vi "Write_setup_to_BSA_F60.vi"(2 "No Of Samples":i32, 3 "Time (s)":sgl, 4 "BSA Setup In":T1={"Wavelength (nm)"=514.5, "Vel Comp"="W", "Max Velocity"=0.0, "Min Velocity"=0.0, "Max Record length"=2, "Signal gain (dB)"=30, "High voltage"=2000, "Optics Conversion Factor"=0.0, "Min Record length"=2, "Multiply Velocity by -1"=FALSE, "Signal to Noise Ratio"="0", "Validation Ratio"="4", "Probe"="", "Laser"="", "BSA"="", "Lense"="", "Beam Separation (mm)"=514.5, "Focal Length (mm)"=514.5, "COLOUR"=52224, "BSA IP"="", "Velocity Range (m/s)"=0.0, "Centre Velocity (m/s)"=0.0, "Unshifted mW"=0.0, "Shifted mW"=0.0, "Bandwidth Hz"=0.0, "Req Sampling Rate Hz"=100.0, "Ch"=0, "CenterFreq Hz"=0.0, "Laser IP"=""} {"Req Sampling Rate Hz" min=1.0; "Shifted mW" format="%.1g"; "Unshifted mW" format="%.1g"; "Centre Velocity (m/s)" format="%.2g"; "Velocity Range (m/s)" format="%.2g"; "Focal Length (mm)" format="%.1f"; "Beam Separation (mm)" format="%.1f"; "Optics Conversion Factor" format="%.3g"; "High voltage" min=0 max=2040 step=8; "Signal gain (dB)" min=0 max=30 step=1; "Min Velocity" format="%.2g"; "Max Velocity" format="%.2g"; "Wavelength (nm)" format="%.1f"}, 5 "BSA":refnum<k7>) -> (0 "error out":errorcluster, 1 "reference out":refnum<k7>)   [LabVIEW 2020]
uses:
  LDA_Channel.ctl
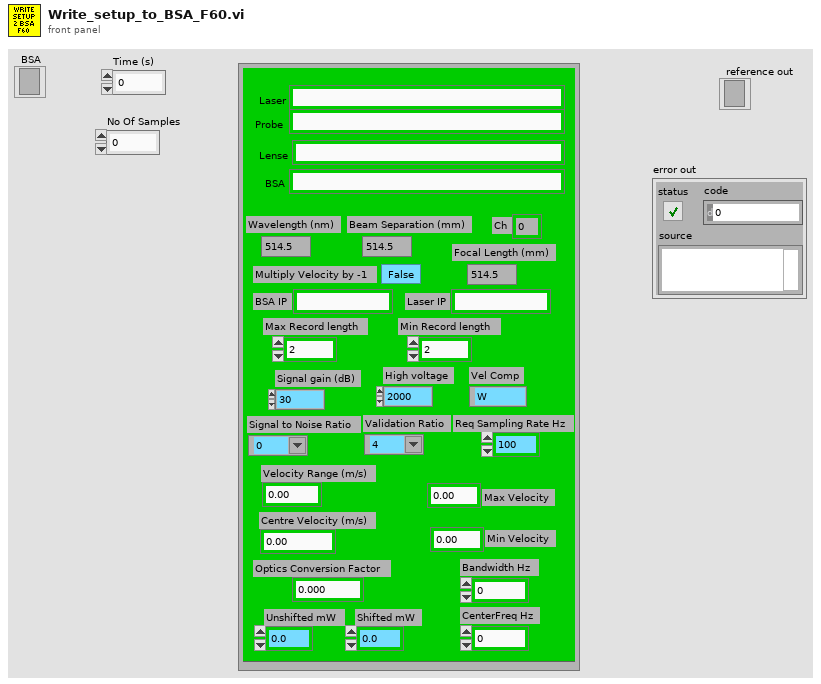
[diagram p1: front panel]
types:
  T1 = typedef "LDA_Channel.ctl" = cluster{"Wavelength (nm)":dbl, "Vel Comp":string, "Max Velocity":dbl, "Min Velocity":dbl, "Max Record length":u16, "Signal gain (dB)":i16, "High voltage":i16, "Optics Conversion Factor":dbl, "Min Record length":u16, "Multiply Velocity by -1":bool, "Signal to Noise Ratio":string, "Validation Ratio":string, "Probe":string, "Laser":string, "BSA":string, "Lense":string, "Beam Separation (mm)":dbl, "Focal Length (mm)":dbl, "COLOUR":u32, "BSA IP":string, "Velocity Range (m/s)":dbl, "Centre Velocity (m/s)":dbl, "Unshifted mW":dbl, "Shifted mW":dbl, "Bandwidth Hz":dbl, "Req Sampling Rate Hz":dbl, "Ch":i32, "CenterFreq Hz":dbl, "Laser IP":string}
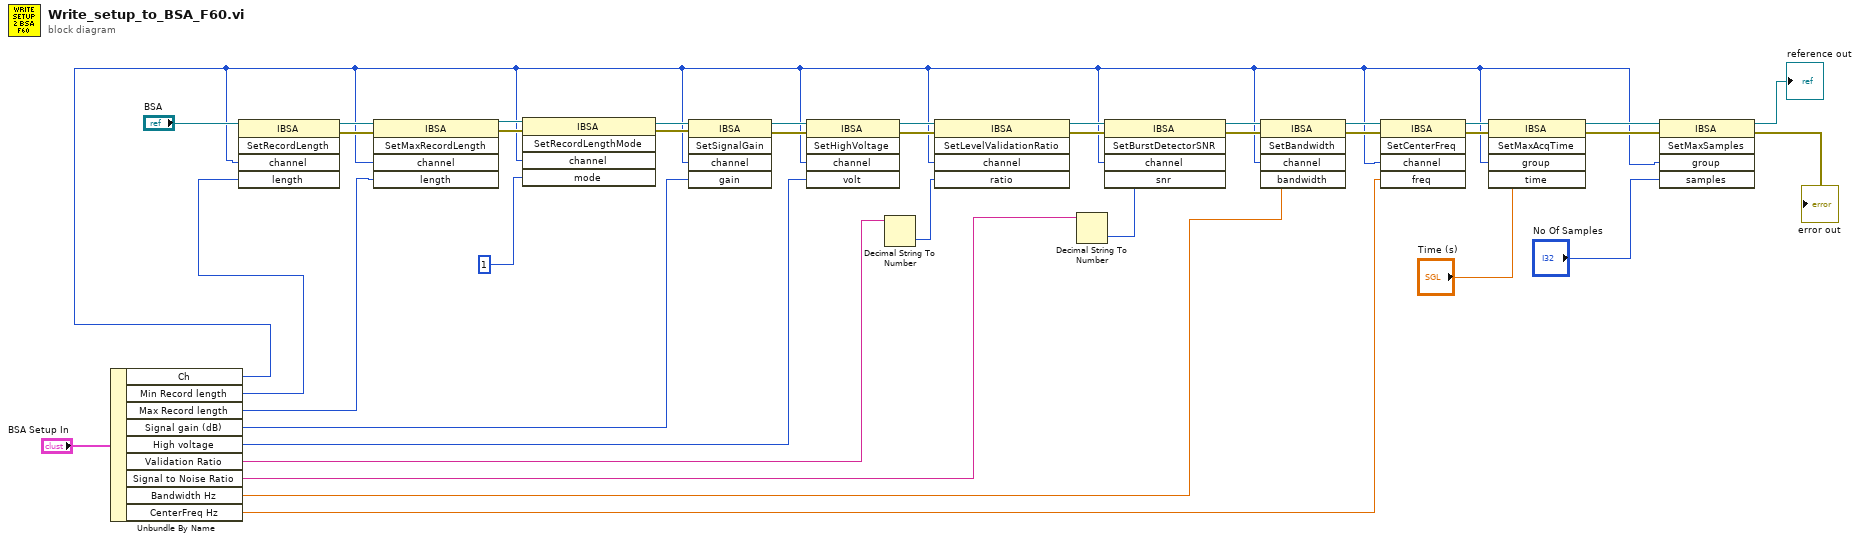
[diagram p0: block diagram]
diagram:
  n1 = Unbundle By Name("BSA Setup In") -> ("Ch"=w1:i32, "Min Record length"=w4:u16, "Max Record length"=w3:u16, "Signal gain (dB)"=w20:i16, "High voltage"=w19:i16, "Validation Ratio"=w18:string, "Signal to Noise Ratio"=w15:string, "Bandwidth Hz"=w14:dbl, "CenterFreq Hz"=w13:dbl)
  n2 = invoke class="IBSA" method="SetRecordLength"(reference="BSA", "channel"=w1, "length"=w4) -> (reference out=w37:refnum<k7>, error out=w26:errorcluster)  [unwired: 2 in, 3 out]
  n3 = invoke class="IBSA" method="SetMaxRecordLength"(reference=w37, error in=w26, "channel"=w1, "length"=w3) -> (reference out=w25:refnum<k7>, error out=w24:errorcluster)  [unwired: 1 in, 3 out]
  n4 = invoke class="IBSA" method="SetRecordLengthMode"(reference=w25, error in=w24, "channel"=w1, "mode"=1) -> (reference out=w23:refnum<k7>, error out=w22:errorcluster)  [unwired: 1 in, 3 out]
  n5 = invoke class="IBSA" method="SetSignalGain"(reference=w23, error in=w22, "channel"=w1, "gain"=w20) -> (reference out=w36:refnum<k7>, error out=w27:errorcluster)  [unwired: 1 in, 3 out]
  n6 = invoke class="IBSA" method="SetHighVoltage"(reference=w36, error in=w27, "channel"=w1, "volt"=w19) -> (reference out=w35:refnum<k7>, error out=w28:errorcluster)  [unwired: 1 in, 3 out]
  n7 = Decimal String To Number(string=w18) -> (number=w17:i32)  [unwired: 3 out]
  n8 = invoke class="IBSA" method="SetLevelValidationRatio"(reference=w35, error in=w28, "channel"=w1, "ratio"=w17) -> (reference out=w34:refnum<k7>, error out=w29:errorcluster)  [unwired: 1 in, 3 out]
  n9 = Decimal String To Number(string=w15) -> (number=w16:i32)  [unwired: 3 out]
  n10 = invoke class="IBSA" method="SetBurstDetectorSNR"(reference=w34, error in=w29, "channel"=w1, "snr"=w16) -> (reference out=w33:refnum<k7>, error out=w30:errorcluster)  [unwired: 1 in, 3 out]
  n11 = invoke class="IBSA" method="SetBandwidth"(reference=w33, error in=w30, "channel"=w1, "bandwidth"=w14) -> (reference out=w32:refnum<k7>, error out=w31:errorcluster)  [unwired: 1 in, 3 out]
  n12 = invoke class="IBSA" method="SetCenterFreq"(reference=w32, error in=w31, "channel"=w1, "freq"=w13) -> (reference out=w10:refnum<k7>, error out=w9:errorcluster)  [unwired: 1 in, 3 out]
  n13 = invoke class="IBSA" method="SetMaxAcqTime"(reference=w10, error in=w9, "group"=w1, "time"="Time (s)") -> (reference out=w11:refnum<k7>, error out=w12:errorcluster)  [unwired: 1 in, 3 out]
  n14 = invoke class="IBSA" method="SetMaxSamples"(reference=w11, error in=w12, "group"=w1, "samples"="No Of Samples") -> (reference out=→"reference out":refnum<k7>, error out=→"error out":errorcluster)  [unwired: 1 in, 3 out]
